vi "Create.vi"(8 "error in (no error)":errorcluster, 11 "I32 in":i32) -> (0 "error out":errorcluster, 3 "Int32 out":refnum<class "Int32.lvclass">)   [LabVIEW 2013, in "MDSplus.lvlib" / "Int32.lvclass"]
uses:
  <vilib>/MDSplus/Classes/Data_Class/Scalar_Class/Int32_Class/Int32.lvclass
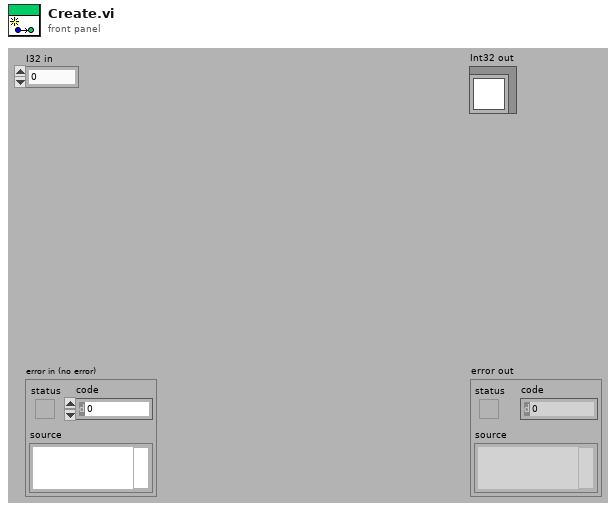
[diagram p1: front panel]
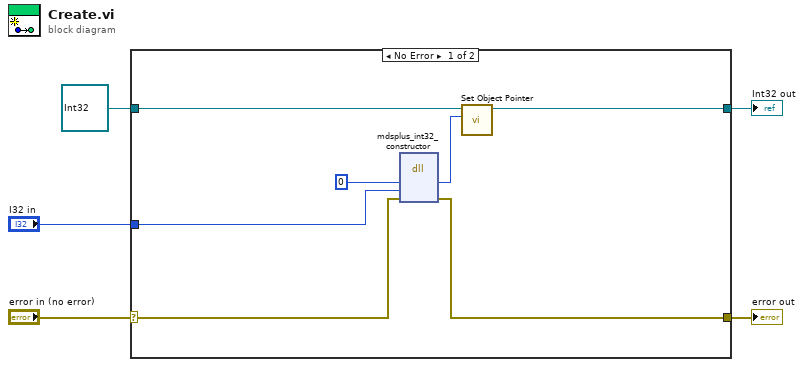
[diagram p0: block diagram]
diagram:
  n1 = case shown="No Error" "error in (no error)" {
    selector: "error in (no error)" -> [w10 w14]
    tunnel: [w6 w14] -> w4
    tunnel: [w7 w13] -> w2
    tunnel: refnum<class "Int32.lvclass"> refnum ("Float32 in") -> [w8 w13]
    tunnel: "I32 in" -> [w9 _]
    frame No Error {
      n2 = dll-call lib="MDSobjectsLVShr" fn="mdsplus_int32_constructor"("lvInt32PtrOut"=i64 0 ("lvTreePtr"), "valIn"=w9, "error"=w10) -> ("lvInt32PtrOut"=w11:i64, "error"=w6:errorcluster)  [unwired: 5 in, 2 out]
      n3 = call-dynamic "Set Object Pointer.vi"("Object Pointer"=w11, "Data in"=w8) -> ("Data out"=w7:refnum<class "Int32.lvclass">)  [unwired: 9 in]
    }
    frame Error {
    }
  }
  "error out" <- w4
  "Int32 out" <- w2
